vi "DAQmx Create Channel (AI-Temperature-Built-in Sensor).vi"(0 "task in":refnum<k21>, 5 "physical channels":tag, 7 "name to assign":string, 9 "units":i32(ring)=10143 items=["Deg C"=10143, "Deg F"=10144, "Kelvins"=10325, "Deg R"=10145, "From Custom Scale"=10065], 11 "error in":errorcluster) -> (4 "task out":refnum<k21>, 15 "error out":errorcluster)   [LabVIEW 2020]
doc: "Creates channel(s) that use the built-in sensor of a terminal block or device to measure temperature. On SCXI modules, for example, the built-in sensor could be the CJC sensor."
uses:
  nilvaiu.dll
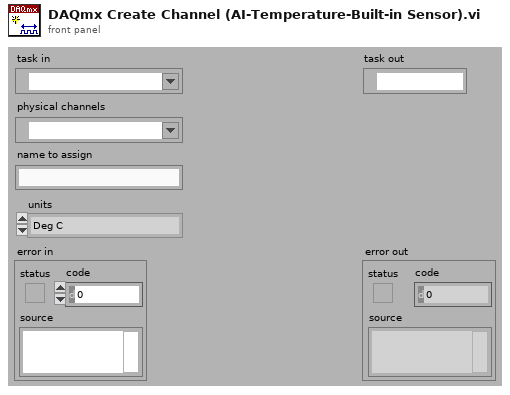
[diagram p1: front panel]
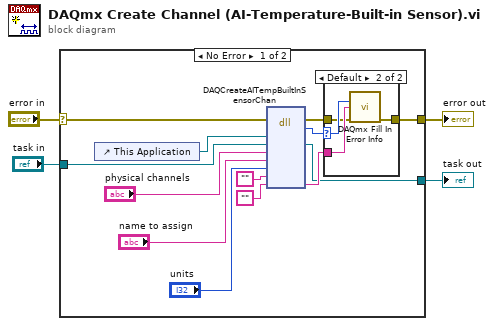
[diagram p0: block diagram]
diagram:
  n1 = case shown="No Error" "error in" {
    selector: "error in" -> [w7 w23]
    tunnel: "task in" -> [w10 w24]
    tunnel: [w9 w23] -> w3
    tunnel: [w8 w24] -> w2
    frame No Error {
      n2 = control-ref of="This Application"() -> (w11:refnum<vi>)
      n3 = dll-call lib="nilvaiu.*" fn="DAQCreateAITempBuiltInSensorChan"(error in=w7, "lvAppRef"=w11, "refObjPtr"=w10, "physicalChannelName"="physical channels", "channelNameIn"="name to assign", "units"="units", "channelNamesOut"="", "extendedErrorInfo"="") -> (error out=w17:errorcluster, "return type"=w16:i32, "refObjPtr"=w8:refnum<k21>, "extendedErrorInfo"=w15:string)  [unwired: 7 in, 1 out]
      n4 = case shown="Default" w16 {
        selector: w16 -> [_ w21]
        tunnel: w17 -> [w18 w19]
        tunnel: [w18 w22] -> w9
        tunnel: w15 -> [_ w20]
        frame 0 {
        }
        frame Default {
          n5 = call "DAQmx Fill In Error Info.vi"("status code"=w21, "extended error info"=w20, "error in"=w19) -> ("error out"=w22:errorcluster)  [unwired: 1 in, 11 out]
        }
      }
    }
    frame Error {
    }
  }
  "task out" <- w2
  "error out" <- w3
